vi "set_origin.vi"(8 "error in (no error)":errorcluster, 11 "StageMH110930Scientifica in":refnum<class "StageMH110930Scientifica.lvclass">) -> (0 "error out":errorcluster, 3 "StageMH110930Scientifica out":refnum<class "StageMH110930Scientifica.lvclass">)   [LabVIEW 2010, in "StageMH110930Scientifica.lvclass"]
uses:
  StageMH110930Scientifica.lvclass
  StageDL090409Scaffold/StageDL090409Scaffold/StageDL090409Scaffold.lvclass
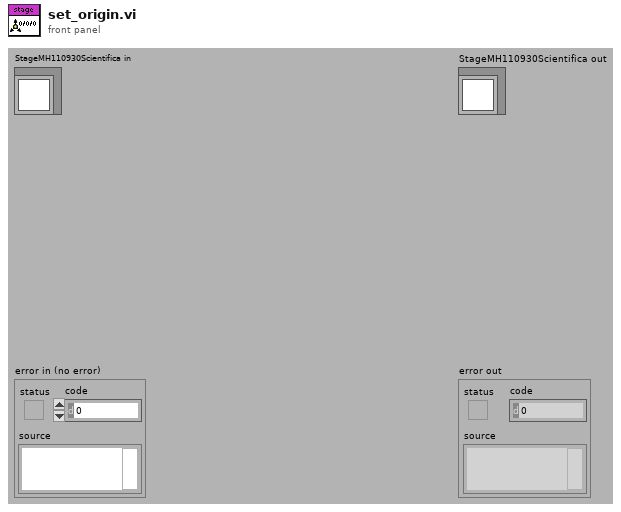
[diagram p1: front panel]
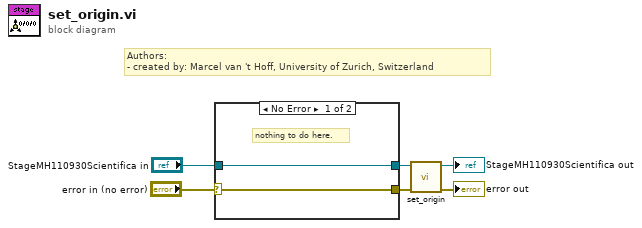
[diagram p0: block diagram]
diagram:
  # "Authors: \n- created by: Marcel van 't Hoff, University of Zurich, Switzerland"
  n1 = case shown="No Error" "error in (no error)" {
    selector: "error in (no error)" -> [w7 w10]
    tunnel: [w7 w10] -> w3
    tunnel: "StageMH110930Scientifica in" -> [w8 w9]
    tunnel: [w8 w9] -> w1
    frame No Error {
      # "nothing to do here."
    }
    frame Error {
    }
  }
  n2 = call-parent "set_origin.vi"("error in (no error)"=w3, "StageDL090409Scaffold in"=w1) -> ("error out"=→"error out":errorcluster, "StageDL090409Scaffold out"=→"StageMH110930Scientifica out":refnum<class "StageMH110930Scientifica.lvclass">)  [unwired: 8 in]
